vi "SetDUTRefValue.vi"(10 "DUTValue":T1={"测试时间"=0.0, "电源开关"=FALSE, "SN"="", "开始按钮"=FALSE, "StopTest"=FALSE, "通信信息"="", "测试状态"="READY", "测试项目栏"=1, "测试结果"={"电流"=FALSE, "SD卡"=FALSE, "USB"=FALSE, "收音机"=FALSE, "DVD"=FALSE, "蓝牙"=FALSE, "IPOD"=FALSE, "终端"=FALSE, "数字电视"=FALSE, "AuxIn"=FALSE, "按键"=FALSE, "ILL检测"=FALSE, "刹车检测"=FALSE, "倒车检测"=FALSE, "方控"=FALSE, "导航"=FALSE, "USB1"=FALSE}, "进度条"=0} {"进度条" scale=0.0..100.0; "测试时间" format="%.1f"}, 11 "DUTRef":refnum<vi>) -> ()   [LabVIEW 2013]
uses:
  Controls/SoltUI.ctl
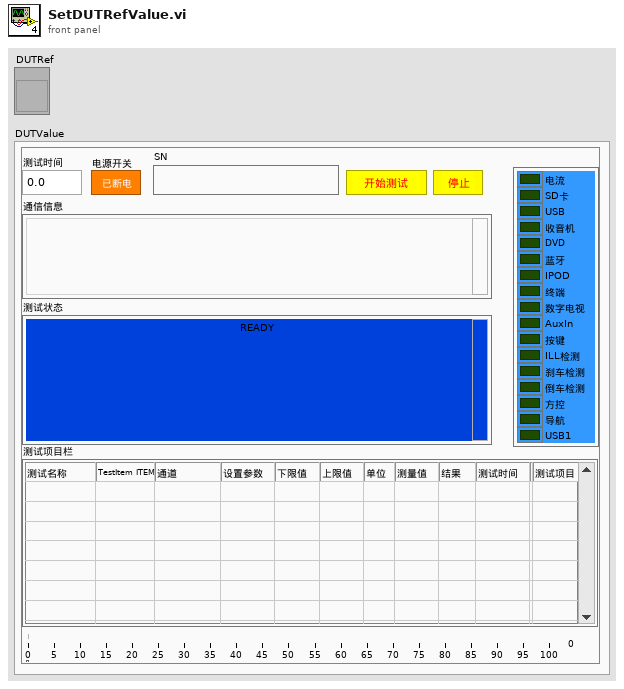
[diagram p1: front panel]
types:
  T1 = typedef "SoltUI.ctl" = cluster{"测试时间":dbl, "电源开关":bool, "SN":string, "开始按钮":bool, "StopTest":bool, "通信信息":string, "测试状态":string, "测试项目栏":i32, "测试结果":cluster{"电流":bool, "SD卡":bool, "USB":bool, "收音机":bool, "DVD":bool, "蓝牙":bool, "IPOD":bool, "终端":bool, "数字电视":bool, "AuxIn":bool, "按键":bool, "ILL检测":bool, "刹车检测":bool, "倒车检测":bool, "方控":bool, "导航":bool, "USB1":bool}, "进度条":i32}
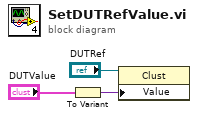
[diagram p0: block diagram]
diagram:
  n1 = To Variant(anything="DUTValue") -> (Variant=w2:variant)
  n2 = property class="Clust"(reference="DUTRef", "Value"=w2) -> ()  [unwired: 1 in, 2 out]
